vi "instance count allowed.vi"(8 "error in":errorcluster, 11 "E2E configuration in":refnum<class "E2E Tag Exchange configuration.lvclass">) -> (0 "error out":errorcluster, 2 "instances allowed":i32, 3 "E2E configuration out":refnum<class "E2E Tag Exchange configuration.lvclass">)   [LabVIEW 2015, in "E2E Tag Exchange configuration.lvclass"]
uses:
  E2E Tag Exchange configuration.lvclass
  E2E Tag Exchange configuration.lvclass/E2E Tag Exchange configuration.ctl
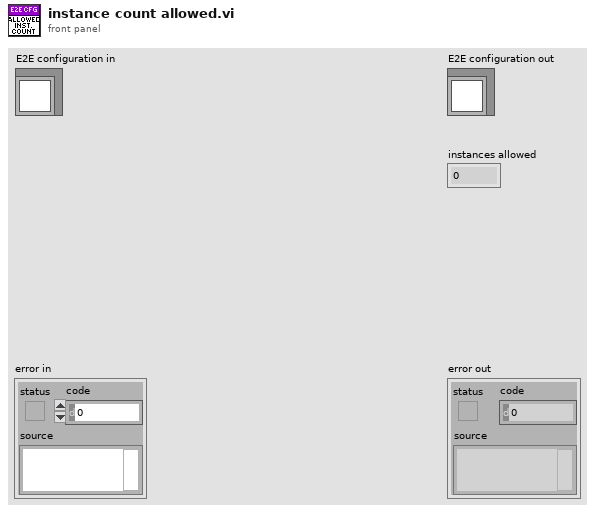
[diagram p1: front panel]
types:
  T1 = typedef "E2E Tag Exchange configuration.lvclass/Runtime Implementation.ctl" = enum16{"RT FIFO", "UDP"}
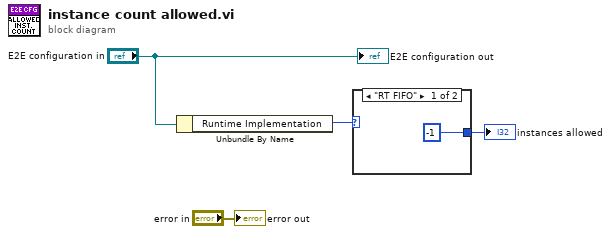
[diagram p0: block diagram]
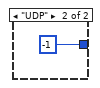
[diagram p2: hidden frame]
diagram:
  n1 = Unbundle By Name("E2E configuration in") -> ("Runtime Implementation"=w2:T1)
  n2 = case shown="\"RT FIFO\"" w2 {
    tunnel: [-1 ("instances allowed") -1 ("instances allowed")] -> w1
    frame "RT FIFO" {
    }
    frame "UDP" {
    }
  }
  "instances allowed" <- w1
  "error out" <- "error in"
  "E2E configuration out" <- "E2E configuration in"
